vi "HH_Go2XYZ.vi"() -> ()   [LabVIEW 2016]
panel:
  out "error out":errorcluster
  out "Initial Position":T1
  out "Final Position":T2
  in  "Go To Coordinates":T3={"Go to X"=150.0, "Go to Y"=100.0, "Go to Z"=25.0}
  in  "Axes Speeds":T4={"X Speed"=25.0, "Y Speed"=12.5, "Z Speed"=5.0}
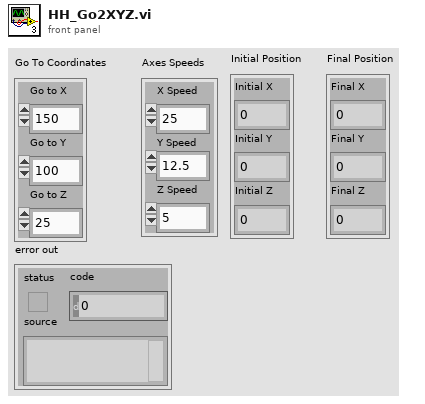
[diagram p1: front panel]
types:
  T1 = cluster{"Initial X":dbl, "Initial Y":dbl, "Initial Z":dbl}
  T2 = cluster{"Final X":dbl, "Final Y":dbl, "Final Z":dbl}
  T3 = cluster{"Go to X":dbl, "Go to Y":dbl, "Go to Z":dbl}
  T4 = cluster{"X Speed":dbl, "Y Speed":dbl, "Z Speed":dbl}
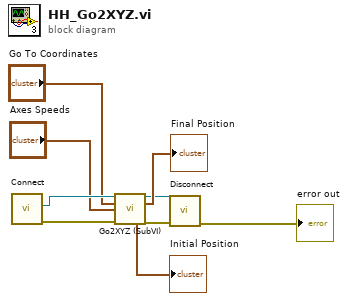
[diagram p0: block diagram]
diagram:
  n1 = call "Connect.vi"() -> ("error out"=w8:errorcluster, "controller"=w9:refnum<k24>)  [unwired: 10 in]
  n2 = call "Go2XYZ (SubVI).vi"(".NET Refnum in"=w9, "Go to Coordinates"="Go To Coordinates", "Axis Speeds"="Axes Speeds", "error in (no error)"=w8) -> (".NET Refnum out"=w2:refnum<k24>, "Final Position"=→"Final Position":T2, "Initial Position"=→"Initial Position":T1, "error out"=w4:errorcluster)  [unwired: 7 in, 1 out]
  n3 = call "Disconnect.vi"("error in (no error)"=w4, "controller"=w2) -> ("error out"=→"error out":errorcluster)  [unwired: 9 in]
